vi "Element.vi"(11 "Task in":refnum<class "Task.lvclass">) -> (2 "Element":refnum<class "Config Element.lvclass">)   [LabVIEW 2020, in "VolatusConfig.lvlib" / "Task.lvclass"]
uses:
  Task.lvclass
  Task.lvclass/Task.ctl
  lv-cdm/CDM-Config/Config Element/Config Element.lvclass
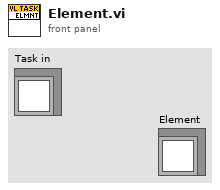
[diagram p1: front panel]
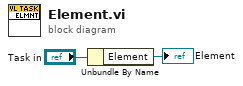
[diagram p0: block diagram]
diagram:
  n1 = Unbundle By Name("Task in") -> ("Element"=→"Element":refnum<class "Config Element.lvclass">)
